vi "Begin.vi"() -> (0 "error out":errorcluster)   [LabVIEW 2013]
doc: "Called before other user functions, this VI is expected to open initial I/O refnums, load in file data, and do all program initialization. Notice that the <B>error out</B> terminal is simply used for data flow. Wiring it to other structures or subVIs ensures that this VI runs first."
uses:
  <vilib>/Rock Robotics/WPI/DriverStation/WPI_DriverStationRobotMode2.ctl
  DBNameEnum.ctl
  <vilib>/Rock Robotics/WPI/SafetyOutput/WPI_SafetyOutputConfigMenu.ctl
  <vilib>/Rock Robotics/WPI/Joystick/WPI_JoystickDeviceEnum.ctl
  RefnameEnum.ctl
  SingleSolenoidAction.ctl
  RollerAction.ctl
  TankDriveAction.ctl
  DoubleSolenoidAction.ctl
  CollectorAction.ctl
  <vilib>/Rock Robotics/SystemInterfaces/Typedef/FPGA_TypedefSolenoidModule.ctl
  <vilib>/Rock Robotics/WPI/Solenoid/WPI_SolenoidChannel.ctl
  <vilib>/Rock Robotics/SystemInterfaces/DIO/FPGA_DIOPWMChannel.ctl
  <vilib>/Rock Robotics/SystemInterfaces/Typedef/FPGA_TypedefDigitalModule.ctl
  <vilib>/Rock Robotics/SystemInterfaces/DIO/FPGA_DIOChannel.ctl
  <vilib>/Rock Robotics/SystemInterfaces/DIO/FPGA_DIORelayChannel.ctl
  <vilib>/Rock Robotics/WPI/Relay/WPI_RelayDirection.ctl
  <vilib>/Rock Robotics/SystemInterfaces/AI/FPGA_AIChannel.ctl
  SonarAction.ctl
  <vilib>/Rock Robotics/SystemInterfaces/Typedef/FPGA_TypedefAnalogModule.ctl
  Example_Code/PressureSensor/PressureSensorAction.ctl
  ServoAction.ctl
  Robot Global Data.vi
  <vilib>/Rock Robotics/WPI/Solenoid/WPI_SolenoidOpenSingle.vi
  <vilib>/Rock Robotics/WPI/MotorControl/WPI_MotorControlOpen Talon.vi
  <vilib>/Rock Robotics/WPI/RobotDrive/WPI_RobotDriveOpen4MotorWithTalon.vi
  <vilib>/Rock Robotics/WPI/Compressor/WPI_CompressorGetSetRefNum.vi
panel:
  in  "Version":string="TF 2.3.2"
  # "SET AS DEFAULT"
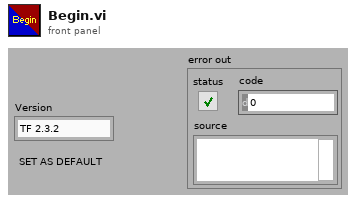
[diagram p1: front panel]
types:
  T1 = typedef "ServoAction.ctl" = enum16{"Init", "SetAngle", "GetAngle", "Disable"}
  T2 = typedef "FPGA_DIOPWMChannel.ctl" = enum8{"PWM 1", "PWM 2", "PWM 3", "PWM 4", "PWM 5", "PWM 6", "PWM 7", "PWM 8", "PWM 9", "PWM 10", "Invalid"}
  T3 = typedef "PressureSensorAction.ctl" = enum16{"Init", "ReadValue", "Disable"}
  T4 = typedef "FPGA_AIChannel.ctl" = enum8{"AI 1", "AI 2", "AI 3", "AI 4", "AI 5", "AI 6", "AI 7", "AI 8", "Invalid"}
  T5 = typedef "FPGA_TypedefAnalogModule.ctl" = enum16{"Analog Module 1", "Analog Module 2"}
  T6 = typedef "FPGA_DIOChannel.ctl" = enum8{"DIO 1", "DIO 2", "DIO 3", "DIO 4", "DIO 5", "DIO 6", "DIO 7", "DIO 8", "DIO 9", "DIO 10", "DIO 11", "DIO 12", "DIO 13", "DIO 14", "Invalid"}
  T7 = typedef "SonarAction.ctl" = enum16{"Init", "ReadValue", "Disable"}
  T8 = typedef "WPI_RelayDirection.ctl" = enum16{"Both directions", "Forward only", "Reverse only"}
  T9 = typedef "FPGA_DIORelayChannel.ctl" = enum8{"Relay 1", "Relay 2", "Relay 3", "Relay 4", "Relay 5", "Relay 6", "Relay 7", "Relay 8", "Invalid"}
  T10 = typedef "WPI_SolenoidChannel.ctl" = enum8{"Solenoid 1", "Solenoid 2", "Solenoid 3", "Solenoid 4", "Solenoid 5", "Solenoid 6", "Solenoid 7", "Solenoid 8", "Invalid"}
  T11 = typedef "FPGA_TypedefSolenoidModule.ctl" = enum16{"Solenoid Module 1", "Solenoid Module 2"}
  T12 = typedef "FPGA_TypedefDigitalModule.ctl" = enum16{"Digital Module 1", "Digital Module 2"}
  T13 = typedef "SingleSolenoidAction.ctl" = enum16{"Init", "SetState", "Disable"}
  T14 = typedef "CollectorAction.ctl" = enum16{"Init", "Raise", "Lower", "Stop", "GetStatus"}
  T15 = typedef "DoubleSolenoidAction.ctl" = enum16{"Init", "Middle", "In", "Out"}
  T16 = typedef "TankDriveAction.ctl" = enum16{"Init", "LinearDrive", "SetValue", "Disable"}
  T17 = typedef "RefnameEnum.ctl" = enum16{"TankDrive", "Controller1", "Controller2", "SonicShifter", "Compressor"}
  T18 = typedef "RollerAction.ctl" = enum16{"Init", "Off", "Forward", "Reverse"}
  T19 = typedef "WPI_JoystickDeviceEnum.ctl" = enum16{"USB 1", "USB 2", "USB 3", "USB 4", "Kinect 1", "Kinect 2"}
  T20 = typedef "WPI_SafetyOutputConfigMenu.ctl" = enum16{"Enable", "Disable"}
  T21 = typedef "DBNameEnum.ctl" = enum16{"Version"}
  T22 = typedef "WPI_DriverStationRobotMode2.ctl" = enum16{"Autonomous Disabled", "Autonomous Enabled", "Teleop Disabled", "Teleop Enabled", "Timeout", "Finish", "Test Disabled", "Test Enabled"}
  T23 = typedef "WPI_JoystickDevRef.ctl" = cluster{"Device":T19}
  T24 = typedef "WPI_RobotDriveDevRef.ctl" = cluster{"DevStatus":errorcluster, "Motors[]":T25[], "Square Inputs":bool, "Max Output":dbl, "Isochronous":bool}
  T25 = typedef "WPI_MotorControlDeviceRef.ctl" = cluster{"DeviceStatus":errorcluster, "Type":enum16{"PWM", "CAN"}, "PWM":cluster{"Digital Module":T12, "PWM Channel":T2, "DeadBand":T26}, "CAN":cluster{"Device Number":u8, "Control Mode":T27, "Semaphore":T28, "Max Vout":dbl}, "Invert":bool, "TransformRef":T29, "InvTransformRef":T29}
  T26 = typedef "WPI_PWMDeadband.ctl" = cluster{"Name":string, "maxPositivePwm":i32, "minPositivePwm":i32, "centerPwm":i32, "maxNegativePwm":i32, "minNegativePwm":i32, "angularRange":u16}
  T27 = typedef "WPI_CANJaguar_ControlMode.ctl" = enum8{"Percent VBus", "Current", "Speed", "Position", "Voltage"}
  T28 = typedef "Semaphore RefNum" = refnum<k1>
  T29 = typedef "WPI_PWMTransform_ConPane.ctl" = refnum<vi>
  T30 = typedef "WPI_SolenoidDevRef.ctl" = cluster{"DevStatus":errorcluster, "Solenoid Module":T11, "Forward Solenoid Channel":T10, "Reverse Solenoid Channel":T10}
  T31 = typedef "WPI_AnalogChannelDevRef.ctl" = cluster{"DevStatus":errorcluster, "Analog Module":T5, "Analog Channel":T4}
  T32 = typedef "WPI_DigitalInputDevRef.ctl" = cluster{"DevStatus":errorcluster, "DIO Channel":T6, "Digital Module":T12}
  T33 = typedef "WPI_CompressorDevRef.ctl" = cluster{"DevStatus":errorcluster, "DigitalInputDevRef":T32, "RelayDevRef":T34}
  T34 = typedef "WPI_RelayDevRef.ctl" = cluster{"DevStatus":errorcluster, "Relay Channel":T9, "Digital Module":T12, "Relay Direction":T8}
  T35 = typedef "WPI_ServoDeviceRef.ctl" = cluster{"DeviceStatus":errorcluster, "Digital Module":T12, "PWM Channel":T2, "DeadBand":T26}
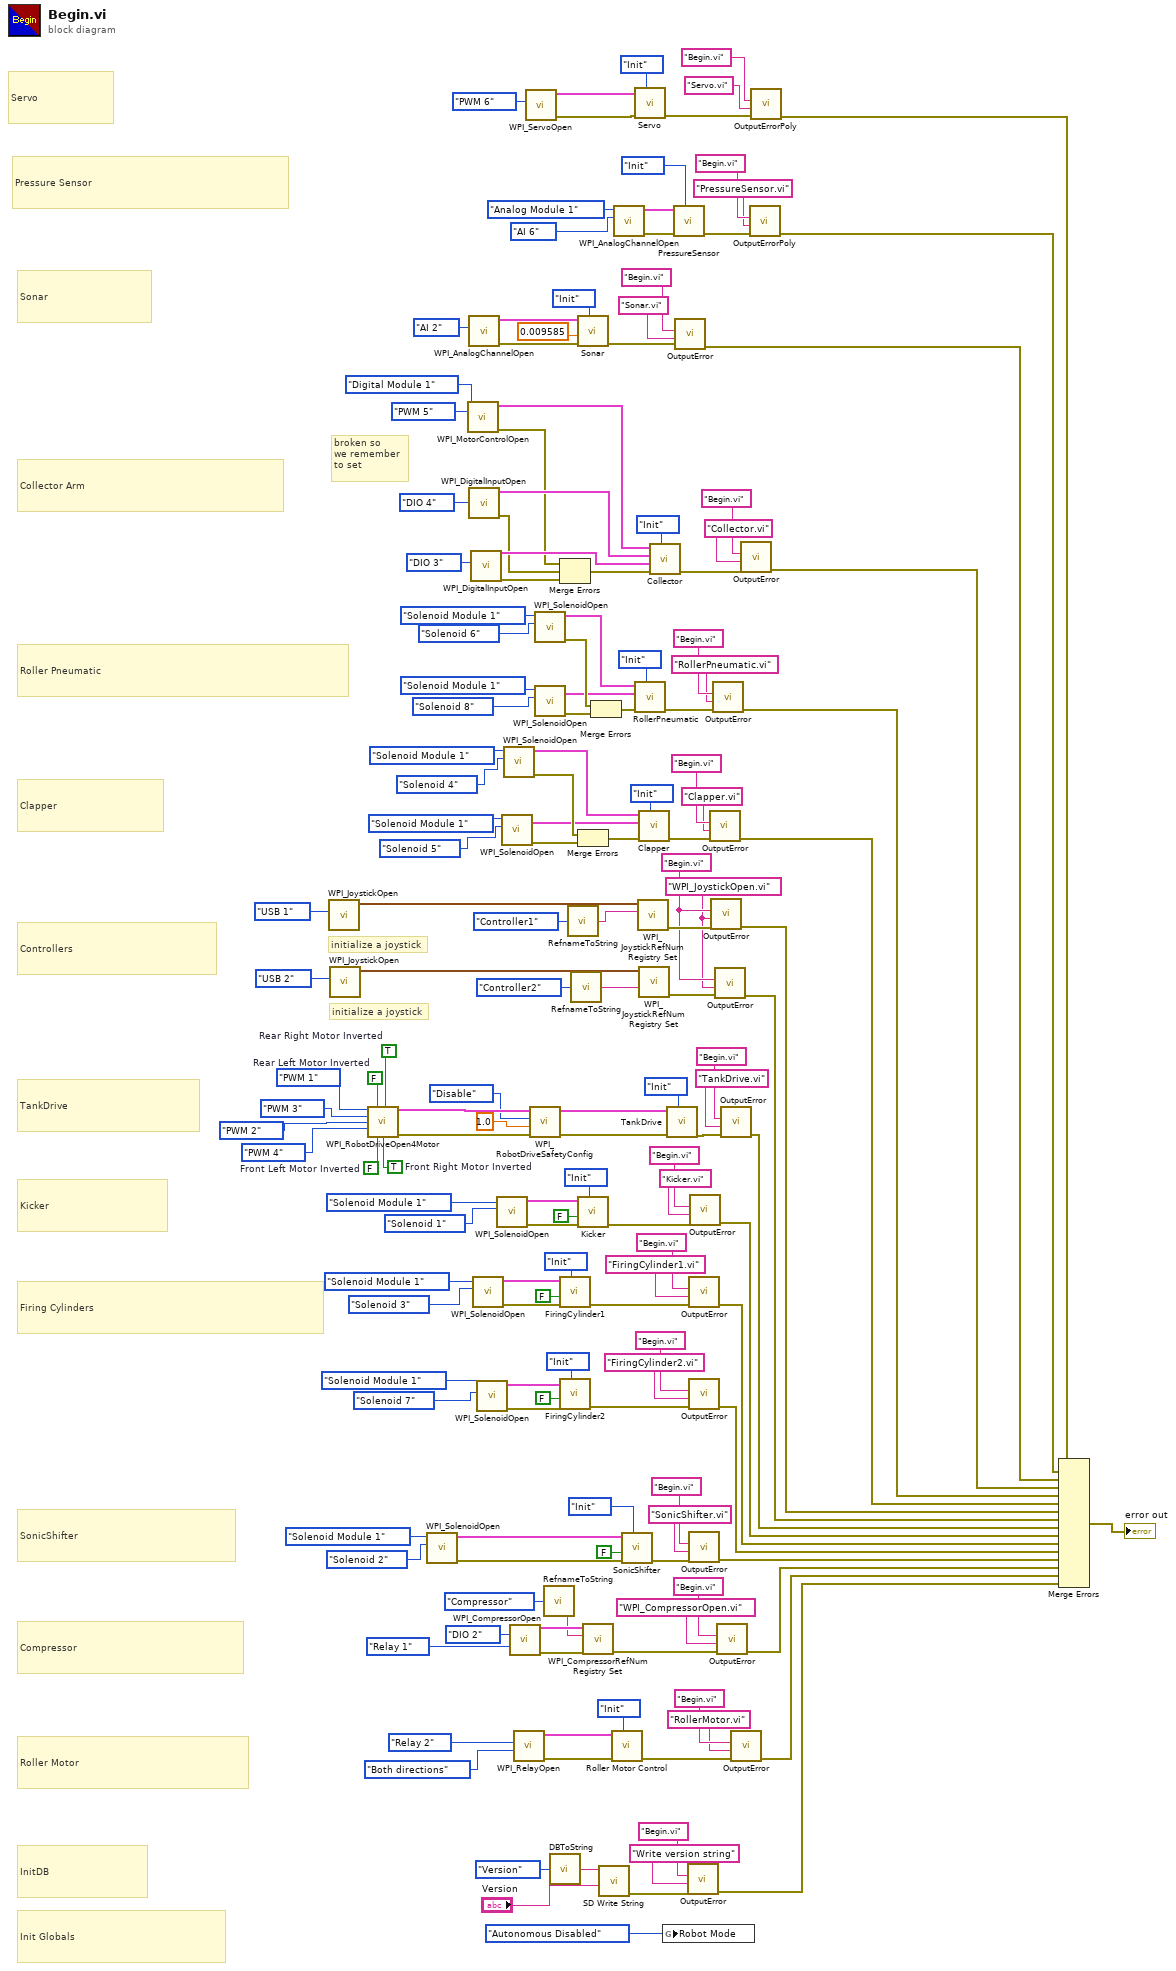
[diagram p0: block diagram]
diagram:
  w22 = TRUE  # Front Right Motor Inverted
  w23 = FALSE  # Front Left Motor Inverted
  w24 = TRUE  # Rear Right Motor Inverted
  w25 = FALSE  # Rear Left Motor Inverted
  w152 = "WPI_JoystickOpen.vi" ("Causing VI")
  w153 = "Begin.vi" ("Calling VI")
  # "Servo"
  # "Pressure Sensor"
  # "broken so\nwe remember\nto set"
  # "Sonar"
  # "Collector Arm"
  # "Firing Cylinders"
  # "Roller Pneumatic"
  # "Clapper"
  # "Compressor"
  # "Roller Motor"
  # "SonicShifter"
  # "Controllers"
  # "initialize a joystick"
  # "initialize a joystick"
  # "TankDrive"
  # "Init Globals"
  # "InitDB"
  # "Kicker"
  n1 = call <vilib>:"WPI_JoystickOpen.vi"("JoystickDevice"=WPI_JoystickDeviceEnum."USB 1") -> ("JoystickDevRef"=w161:T23)  [unwired: 10 in]
  n2 = call <vilib>:"WPI_JoystickOpen.vi"("JoystickDevice"=WPI_JoystickDeviceEnum."USB 2") -> ("JoystickDevRef"=w158:T23)  [unwired: 10 in]
  n3 = call-poly <vilib>:"WPI_RobotDriveOpen4Motor.vi"("Rear Left Motor"=FPGA_DIOPWMChannel."PWM 1", "Rear Left Motor Inverted"=w25, "Rear Right Motor Inverted"=w24, "Rear Right Motor"=FPGA_DIOPWMChannel."PWM 3", "Front Left Motor"=FPGA_DIOPWMChannel."PWM 2", "Front Right Motor"=FPGA_DIOPWMChannel."PWM 4", "Front Left Motor Inverted"=w23, "Front Right Motor Inverted"=w22) -> ("RobotDriveDevRef"=w166:T24, "error out"=w165:errorcluster)  [unwired: 6 in]
  n4 = call-poly <vilib>:"WPI_SolenoidOpen.vi"("Solenoid Channel"=WPI_SolenoidChannel."Solenoid 2", "Solenoid Module (Module 1)"=FPGA_TypedefSolenoidModule."Solenoid Module 1") -> ("error out"=w108:errorcluster, "SolenoidDevRef"=w107:T30)  [unwired: 8 in]
  n5 = call-poly <vilib>:"WPI_MotorControlOpen.vi"("PWM Channel"=FPGA_DIOPWMChannel."PWM 5", "Digital Module (Module 1)"=FPGA_TypedefDigitalModule."Digital Module 1") -> ("error out"=w83:errorcluster, "MotorControlDeviceRef"=w89:T25)  [unwired: 8 in]
  n6 = call <vilib>:"WPI_AnalogChannelOpen.vi"("Analog Channel"=FPGA_AIChannel."AI 2") -> ("error out"=w37:errorcluster, "AIDeviceRef"=w38:T31)  [unwired: 9 in]
  n7 = call <vilib>:"WPI_DigitalInputOpen.vi"("DIO Channel"=FPGA_DIOChannel."DIO 4") -> ("error out"=w84:errorcluster, "DigitalInputDevRef"=w88:T32)  [unwired: 9 in]
  n8 = call <vilib>:"WPI_DigitalInputOpen.vi"("DIO Channel"=FPGA_DIOChannel."DIO 3") -> ("error out"=w85:errorcluster, "DigitalInputDevRef"=w87:T32)  [unwired: 9 in]
  n9 = call-poly <vilib>:"WPI_SolenoidOpen.vi"("Solenoid Channel"=WPI_SolenoidChannel."Solenoid 3", "Solenoid Module (Module 1)"=FPGA_TypedefSolenoidModule."Solenoid Module 1") -> ("error out"=w98:errorcluster, "SolenoidDevRef"=w97:T30)  [unwired: 8 in]
  n10 = call-poly <vilib>:"WPI_SolenoidOpen.vi"("Solenoid Channel"=WPI_SolenoidChannel."Solenoid 7", "Solenoid Module (Module 1)"=FPGA_TypedefSolenoidModule."Solenoid Module 1") -> ("error out"=w71:errorcluster, "SolenoidDevRef"=w70:T30)  [unwired: 8 in]
  n11 = call-poly <vilib>:"WPI_SolenoidOpen.vi"("Solenoid Channel"=WPI_SolenoidChannel."Solenoid 1", "Solenoid Module (Module 1)"=FPGA_TypedefSolenoidModule."Solenoid Module 1") -> ("error out"=w106:errorcluster, "SolenoidDevRef"=w103:T30)  [unwired: 8 in]
  n12 = call-poly <vilib>:"WPI_SolenoidOpen.vi"("Solenoid Channel"=WPI_SolenoidChannel."Solenoid 5", "Solenoid Module (Module 1)"=FPGA_TypedefSolenoidModule."Solenoid Module 1") -> ("error out"=w63:errorcluster, "SolenoidDevRef"=w62:T30)  [unwired: 8 in]
  n13 = call-poly <vilib>:"WPI_SolenoidOpen.vi"("Solenoid Channel"=WPI_SolenoidChannel."Solenoid 4", "Solenoid Module (Module 1)"=FPGA_TypedefSolenoidModule."Solenoid Module 1") -> ("error out"=w119:errorcluster, "SolenoidDevRef"=w118:T30)  [unwired: 8 in]
  n14 = call <vilib>:"WPI_CompressorOpen.vi"("Pressure Switch DIO Channel"=FPGA_DIOChannel."DIO 2", "Relay Channel"=FPGA_DIORelayChannel."Relay 1") -> ("CompressorDevRef"=w129:T33, "error out"=w128:errorcluster)  [unwired: 3 in, 9 out]
  n15 = call <vilib>:"WPI_RelayOpen.vi"("Relay Direction"=WPI_RelayDirection."Both directions", "Relay Channel"=FPGA_DIORelayChannel."Relay 2") -> ("error out"=w136:errorcluster, "RelayDevRef"=w134:T34)  [unwired: 8 in]
  n16 = call <vilib>:"WPI_ServoOpen.vi"("PWM Channel"=FPGA_DIOPWMChannel."PWM 6") -> ("error out"=w8:errorcluster, "ServoDeviceRef"=w7:T35)  [unwired: 9 in]
  n17 = call <vilib>:"WPI_RobotDriveSafetyConfig.vi"("error in (no error)"=w165, "timeout (s)"=1.0, "mode"=WPI_SafetyOutputConfigMenu."Disable", "RobotDriveDevRef"=w166) -> ("error out"=w9:errorcluster, "RobotDriveDevRef"=w10:T24)  [unwired: 6 in]
  n18 = call-poly <vilib>:"WPI_SolenoidOpen.vi"("Solenoid Channel"=WPI_SolenoidChannel."Solenoid 6", "Solenoid Module (Module 1)"=FPGA_TypedefSolenoidModule."Solenoid Module 1") -> ("error out"=w109:errorcluster, "SolenoidDevRef"=w110:T30)  [unwired: 8 in]
  n19 = call-poly <vilib>:"WPI_SolenoidOpen.vi"("Solenoid Channel"=WPI_SolenoidChannel."Solenoid 8", "Solenoid Module (Module 1)"=FPGA_TypedefSolenoidModule."Solenoid Module 1") -> ("error out"=w58:errorcluster, "SolenoidDevRef"=w57:T30)  [unwired: 8 in]
  n20 = call "RefnameToString.vi"("Enum"=RefnameEnum."Compressor") -> ("Refname"=w125:string)
  n21 = call "DBToString.vi"("Enum"=DBNameEnum."Version") -> ("Refname"=w168:string)
  n22 = Merge Errors(w83, w84, w85) -> (w86:errorcluster)
  n23 = call "FiringCylinder1.vi"("Action"=SingleSolenoidAction."Init", "error in (no error)"=w98, "Default Position"=FALSE, "SolenoidDevRef"=w97) -> ("error out"=w99:errorcluster)  [unwired: 7 in]
  n24 = call "FiringCylinder2.vi"("Action"=SingleSolenoidAction."Init", "error in (no error)"=w71, "Default Position"=FALSE, "SolenoidDevRef"=w70) -> ("error out"=w66:errorcluster)  [unwired: 7 in]
  n25 = call "RefnameToString.vi"("Enum"=RefnameEnum."Controller1") -> ("Refname"=w150:string)
  n26 = call "RefnameToString.vi"("Enum"=RefnameEnum."Controller2") -> ("Refname"=w148:string)
  n27 = call "Sonar.vi"("Action"=SonarAction."Init", "error in (no error)"=w37, "Scaling factor (V/in)"=0.009585, "AIDeviceRef"=w38) -> ("error out"=w33:errorcluster)  [unwired: 6 in, 1 out]
  n28 = Merge Errors(w119, w63) -> (w64:errorcluster)
  n29 = call "Kicker.vi"("Action"=SingleSolenoidAction."Init", "error in (no error)"=w106, "Default Position"=FALSE, "SolenoidDevRef"=w103) -> ("error out"=w105:errorcluster)  [unwired: 7 in]
  n30 = call <vilib>:"WPI_CompressorRefNum Registry Set.vi"("error in (no error)"=w128, "refnum name"=w125, "CompressorDevRef"=w129) -> ("error out"=w127:errorcluster)  [unwired: 7 in, 1 out]
  n31 = Merge Errors(w109, w58) -> (w59:errorcluster)
  n32 = call <vilib>:"SD Write String.vi"("String"="Version", "Name"=w168) -> ("error out"=w145:errorcluster)  [unwired: 8 in, 1 out]
  n33 = call "Roller Motor Control.vi"("Action"=RollerAction."Init" ("RollerState"), "Error in"=w136, "RelayDevRef"=w134) -> ("Error out"=w135:errorcluster)  [unwired: 8 in]
  n34 = call <vilib>:"WPI_AnalogChannelOpen.vi"("Analog Channel"=FPGA_AIChannel."AI 6", "Analog Module (Module 1)"=FPGA_TypedefAnalogModule."Analog Module 1") -> ("error out"=w17:errorcluster, "AIDeviceRef"=w16:T31)  [unwired: 8 in]
  n35 = call "SonicShifter.vi"("Action"=SingleSolenoidAction."Init" ("Mode"), "error in (no error)"=w108, "Default Position"=FALSE, "SolenoidDevRef"=w107) -> ("error out"=w144:errorcluster)  [unwired: 7 in]
  n36 = call "Servo.vi"("Action"=ServoAction."Init", "error in (no error)"=w8, "ServoDeviceRef"=w7) -> ("error out"=w4:errorcluster)  [unwired: 7 in, 1 out]
  n37 = call "RollerPneumatic.vi"("State"=DoubleSolenoidAction."Init", "Error in"=w59, "Plugged"=w57, "Open"=w110) -> ("Error out"=w113:errorcluster)  [unwired: 7 in]
  n38 = call <vilib>:"WPI_JoystickRefNum Registry Set.vi"("refnum name"=w150, "JoystickDevRef"=w161) -> ("error out"=w154:errorcluster)  [unwired: 8 in, 1 out]
  n39 = call "Clapper.vi"("State"=DoubleSolenoidAction."Init", "Error in"=w64, "Plugged"=w62, "Open"=w118) -> ("Error out"=w117:errorcluster)  [unwired: 7 in]
  n40 = call <vilib>:"WPI_JoystickRefNum Registry Set.vi"("refnum name"=w148, "JoystickDevRef"=w158) -> ("error out"=w155:errorcluster)  [unwired: 8 in, 1 out]
  n41 = call "Collector.vi"("Action"=CollectorAction."Init", "Error in"=w86, "BottomLS"=w87, "TopLS"=w88, "Motor"=w89) -> ("Error out"=w91:errorcluster)  [unwired: 4 in, 2 out]
  n42 = global write "Robot Global Data.vi" "Robot Mode"(WPI_DriverStationRobotMode2."Autonomous Disabled" ("Robot Mode")) -> ()
  n43 = call "TankDrive.vi"("DriveAction"=TankDriveAction."Init", "error in (no error)"=w9, "RobotDriveDevRef"=w10) -> ("error out"=w162:errorcluster)  [unwired: 7 in, 1 out]
  n44 = call "PressureSensor.vi"("Action"=PressureSensorAction."Init", "error in (no error)"=w17, "AIDeviceRef"=w16) -> ("error out"=w14:errorcluster)  [unwired: 7 in, 1 out]
  n45 = call "OutputError.vi"("error in (no error)"=w33, "Causing VI"="Sonar.vi", "Calling VI"="Begin.vi") -> ("error out"=w30:errorcluster)  [unwired: 8 in]
  n46 = call "OutputError.vi"("error in (no error)"=w145, "Causing VI"="Write version string", "Calling VI"="Begin.vi") -> ("error out"=w131:errorcluster)  [unwired: 8 in]
  n47 = call "OutputError.vi"("error in (no error)"=w99, "Causing VI"="FiringCylinder1.vi" ("Calling VI"), "Calling VI"="Begin.vi") -> ("error out"=w73:errorcluster)  [unwired: 8 in]
  n48 = call "OutputError.vi"("error in (no error)"=w66, "Causing VI"="FiringCylinder2.vi" ("Calling VI"), "Calling VI"="Begin.vi") -> ("error out"=w65:errorcluster)  [unwired: 8 in]
  n49 = call "OutputError.vi"("error in (no error)"=w144, "Causing VI"="SonicShifter.vi", "Calling VI"="Begin.vi") -> ("error out"=w143:errorcluster)  [unwired: 8 in]
  n50 = call "OutputError.vi"("error in (no error)"=w105, "Causing VI"="Kicker.vi" ("Calling VI"), "Calling VI"="Begin.vi") -> ("error out"=w74:errorcluster)  [unwired: 8 in]
  n51 = call "OutputError.vi"("error in (no error)"=w117, "Causing VI"="Clapper.vi", "Calling VI"="Begin.vi") -> ("error out"=w78:errorcluster)  [unwired: 8 in]
  n52 = call "OutputError.vi"("error in (no error)"=w154, "Causing VI"=w152, "Calling VI"=w153) -> ("error out"=w77:errorcluster)  [unwired: 8 in]
  n53 = call "OutputError.vi"("error in (no error)"=w113, "Causing VI"="RollerPneumatic.vi", "Calling VI"="Begin.vi") -> ("error out"=w79:errorcluster)  [unwired: 8 in]
  n54 = call "OutputError.vi"("error in (no error)"=w155, "Causing VI"=w152, "Calling VI"=w153) -> ("error out"=w76:errorcluster)  [unwired: 8 in]
  n55 = call "OutputError.vi"("error in (no error)"=w127, "Causing VI"="WPI_CompressorOpen.vi", "Calling VI"="Begin.vi") -> ("error out"=w124:errorcluster)  [unwired: 8 in]
  n56 = call "OutputError.vi"("error in (no error)"=w162, "Causing VI"="TankDrive.vi", "Calling VI"="Begin.vi") -> ("error out"=w75:errorcluster)  [unwired: 8 in]
  n57 = call "OutputError.vi"("error in (no error)"=w135, "Causing VI"="RollerMotor.vi", "Calling VI"="Begin.vi") -> ("error out"=w130:errorcluster)  [unwired: 8 in]
  n58 = call "OutputError.vi"("error in (no error)"=w91, "Causing VI"="Collector.vi", "Calling VI"="Begin.vi") -> ("error out"=w80:errorcluster)  [unwired: 8 in]
  n59 = call-poly "OutputErrorPoly.vi"("error in (no error)"=w14, "Causing VI"="PressureSensor.vi", "Calling VI"="Begin.vi") -> ("error out"=w13:errorcluster)  [unwired: 8 in]
  n60 = call-poly "OutputErrorPoly.vi"("error in (no error)"=w4, "Causing VI"="Servo.vi", "Calling VI"="Begin.vi") -> ("error out"=w1:errorcluster)  [unwired: 8 in]
  n61 = Merge Errors(w1, w13, w30, w80, w79, w78, w77, w76, w75, w74, w73, w65, w143, w124, w130, w131) -> (→"error out":errorcluster)
